vi "read caen.vi"(0 "VISA in":refnum<visa-resource-name>, 1 "Extended Delay":bool=TRUE, 11 "error in":errorcluster, 12 "First read time (ms)":u32=310, 13 "Short Loop Read Time (ms)":u32=150) -> (4 "VISA out":refnum<visa-resource-name>, 6 "Read string":string, 8 "Display array":string[][](array[string]), 10 "Location Cluster":T1, 14 "Display string":string, 15 "error out":errorcluster)   [LabVIEW 2018]
uses:
  location cluster.ctl
  <vilib>/Instr/_visa.llb/Select Event Type.ctl
  CAEN globals.vi
panel:
  out "Waveform Chart":i32(graph)
  out "HB":bool
  out "buffer":string
  out "Display":string[][](array[string])
  out "display error":errorcluster
  out "bytes at port":u32
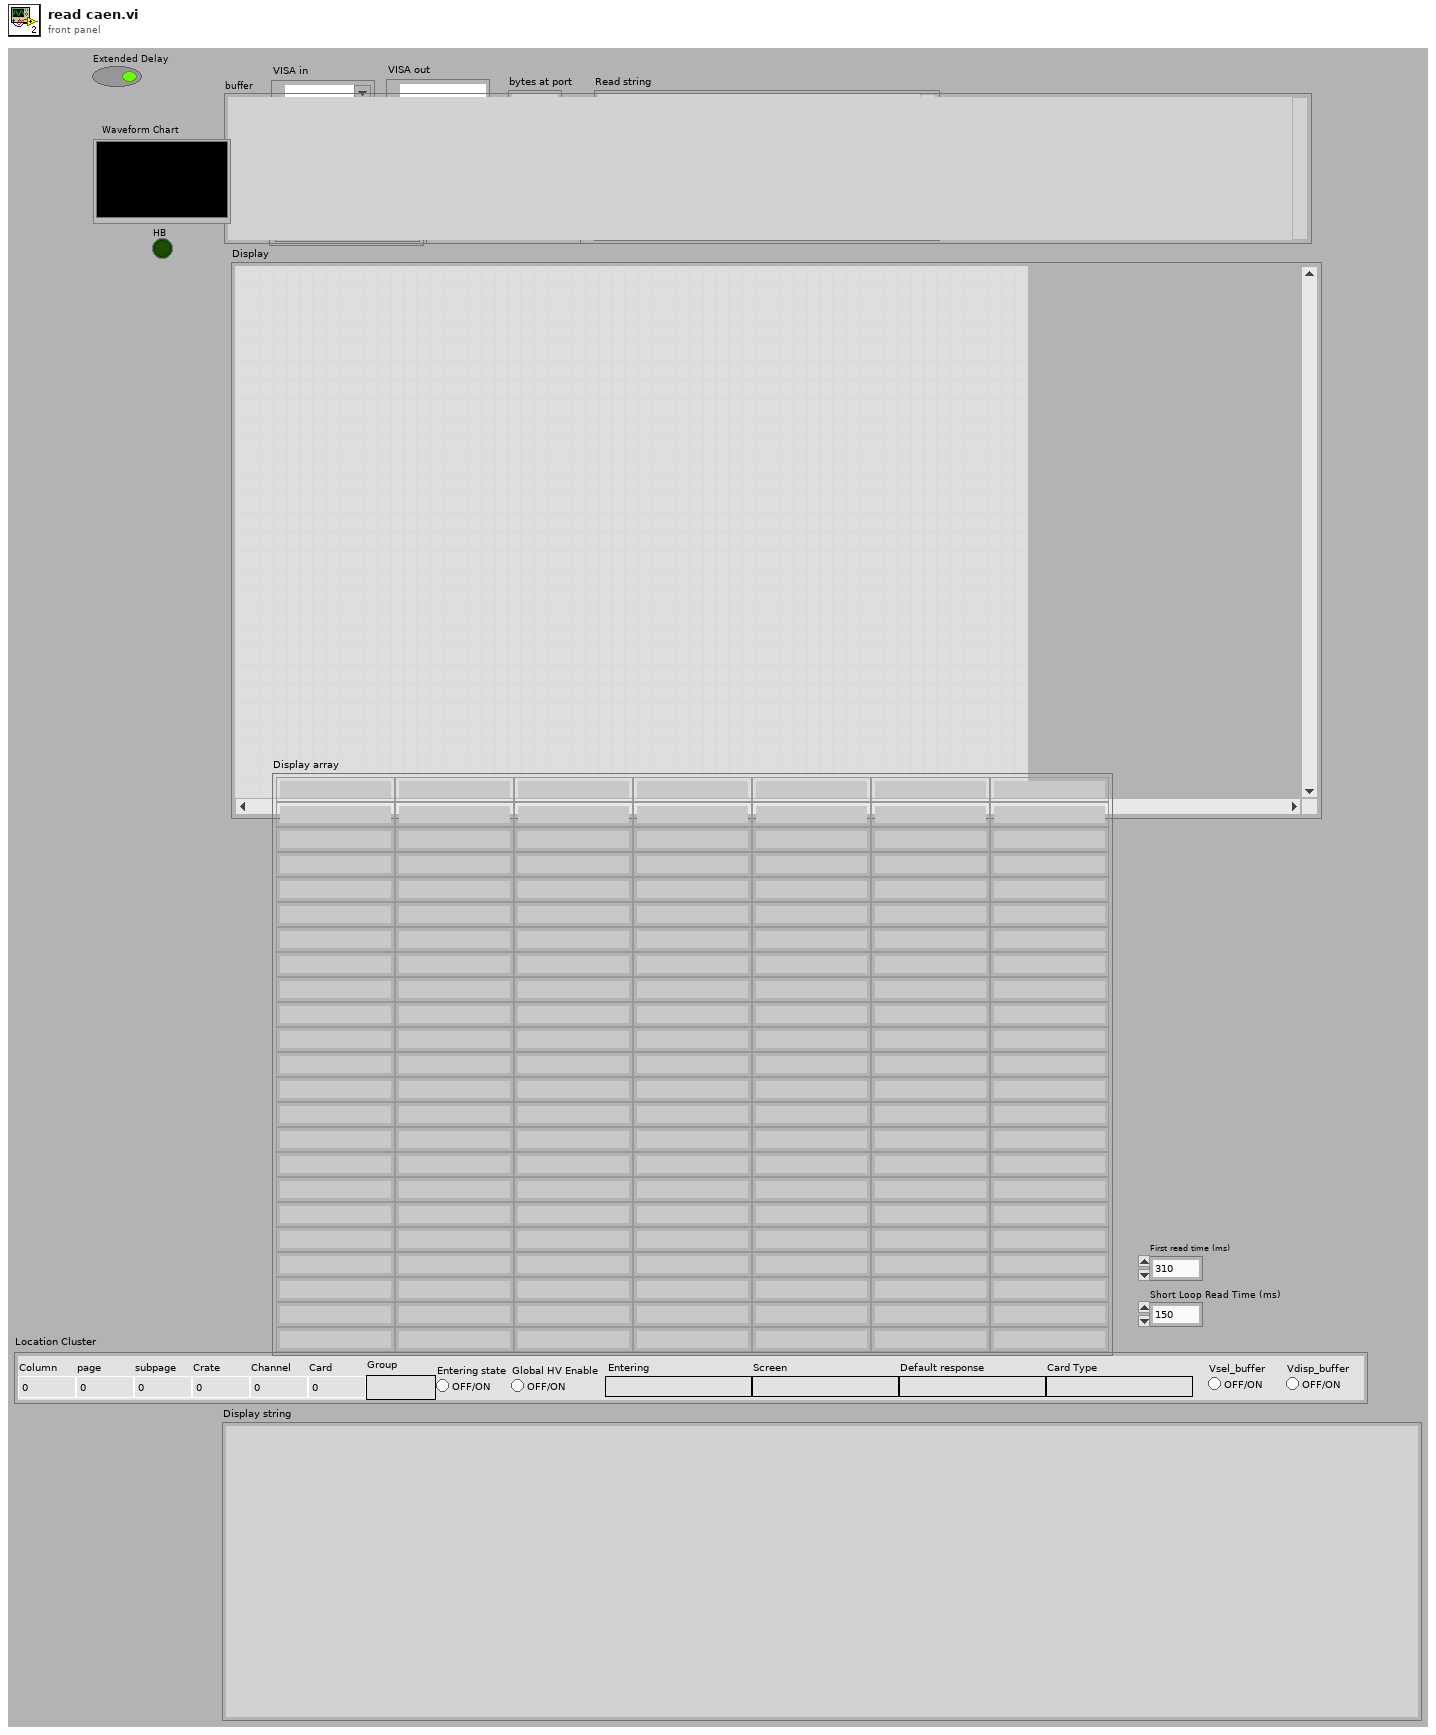
[diagram p1: front panel]
types:
  T1 = typedef "location cluster.ctl" = cluster{"Column":i32, "Card Type":string, "Channel":i32, "Card":i32, "Default response":string, "Entering":string, "Entering state":bool, "subpage":i32, "page":i32, "Crate":i32, "Screen":string, "Group":string, "Global HV Enable":bool, "Vsel_buffer":bool, "Vdisp_buffer":bool}
  T2 = typedef "Select Event Type.ctl" = u32
  T3 = cluster{"Bytes at Port":u32, "Serial Settings:Number of Bytes at Serial Port":u32}
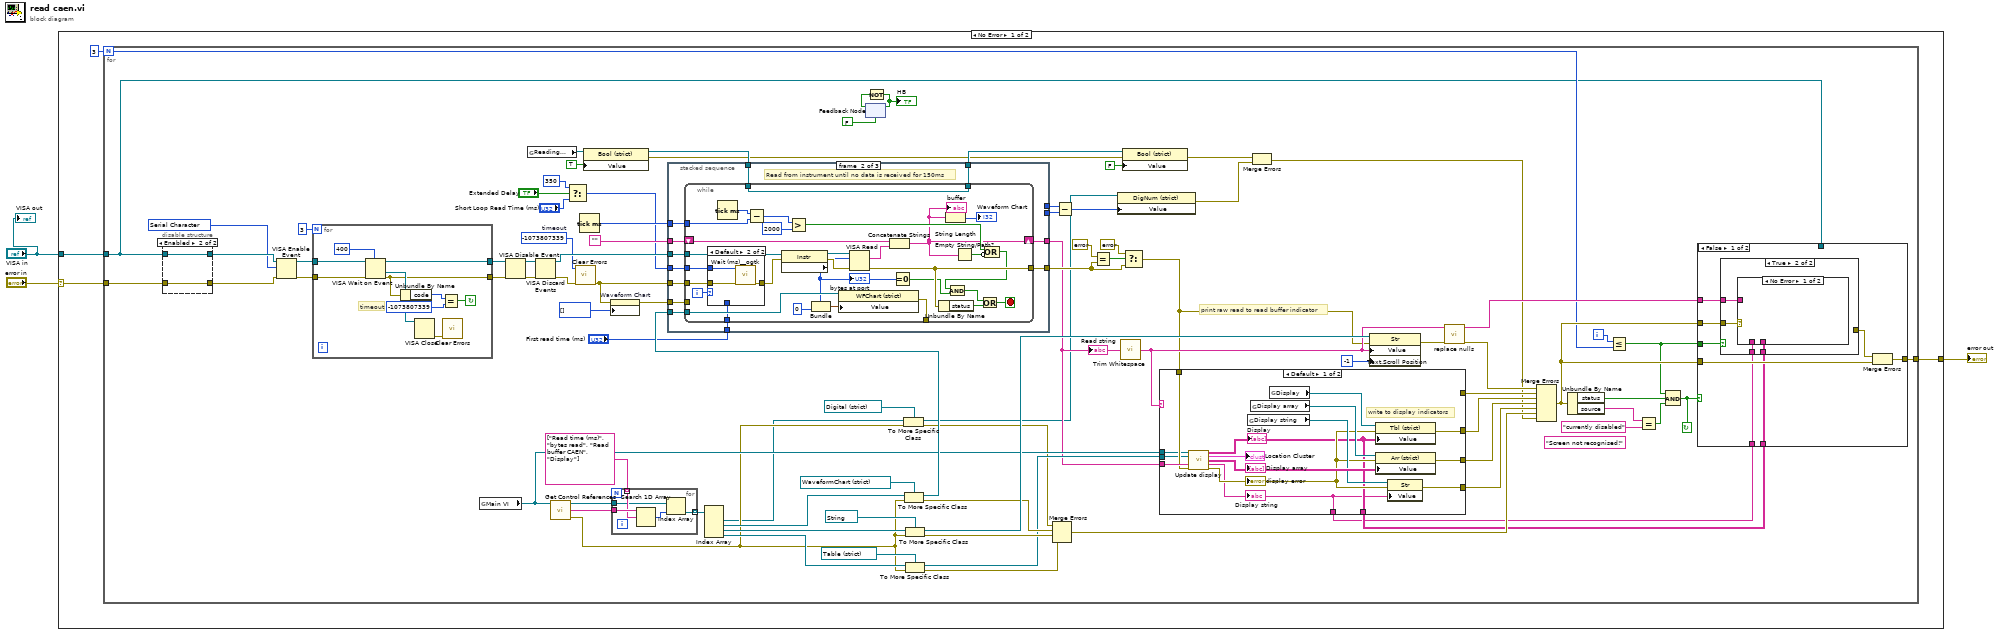
[diagram p0: block diagram]
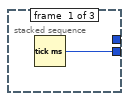
[diagram p2: hidden frame]
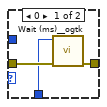
[diagram p3: hidden frame]
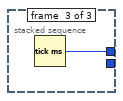
[diagram p4: hidden frame]
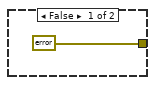
[diagram p5: hidden frame]
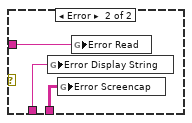
[diagram p6: hidden frame]
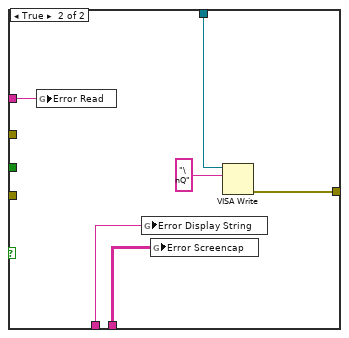
[diagram p7: hidden frame]
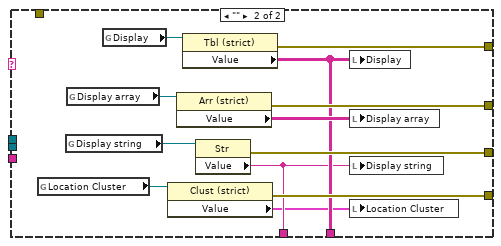
[diagram p8: hidden frame]
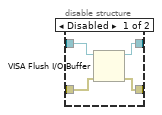
[diagram p9: hidden frame]
diagram:
  n1 = case shown="No Error" "error in" {
    selector: "error in" -> [w4 w218]
    tunnel: [w6 w218] -> w3
    tunnel: "VISA in" -> [w5 _]
    frame No Error {
      n2 = for {
        N: 3 -> [w26]
        tunnel: w4 -> [w74]
        tunnel: w5 -> [w8]
        tunnel: [w47] -> w6
        i -> [w27]
        stop <- w48 continue-if-true
        (unwired) "Screen not recognised!" ("y")
        w35 = -1073807339  # timeout
        w64 = T2 1073684533 items=["Service Request"=1073684491, "Trigger"=3221168138, "Clear"=1073684493, "VXI Signal"=1073684512, "VXI/VME Interrupt"=3221168161, "VXI/VME Sysfail"=1073684509, "VXI/VME Sysreset"=1073684510, "GPIB CIC"=1073684498, "GPIB Talk"=1073684499, "GPIB Listen"=1073684500, "PXI Interrupt"=1073684514, "Serial Break"=1073684515, "Serial TermChar"=1073684516, "Serial CTS"=1073684521, "Serial DSR"=1073684522, "Serial DCD"=1073684524, "Serial RI"=1073684526, "Serial Character"=1073684533, "USB Interrupt"=1073684535, "All Enabled"=1073709055] ("Event Type")
        # "print raw read to read buffer indicator"
        n3 = disable-structure shown="Enabled" {
          disable-tunnel: w8 -> [w210 w212]
          disable-tunnel: w74 -> [w209 w211]
          disable-tunnel: [w208 w212] -> w73
          disable-tunnel: [w207 w211] -> w72
          frame Disabled {
            n4 = VISA Flush I/O Buffer(VISA resource name=w210, error in (no error)=w209) -> (VISA resource name out=w208:refnum<visa-resource-name>, error out=w207:errorcluster)  [unwired: 1 in]
          }
          frame Enabled {
          }
        }
        n5 = VISA Enable Event(8:w72, 10:w64, 11:w73) -> (0:w42:errorcluster, 3:w43:refnum<visa-resource-name>)  [unwired: 1 in]
        n6 = for {
          N: 3 -> [_]
          tunnel: w42 -> [w156]
          tunnel: [w152] -> w37
          tunnel: w43 -> [w157]
          tunnel: [w153] -> w38
          stop <- w149 continue-if-true
          # "timeout"
          n7 = VISA Wait on Event(7:u32 400 ("milliseconds to wait"), 8:w156, 11:w157) -> (0:w152:errorcluster, 1:w155:refnum<visa-resource-name>, 3:w153:refnum<visa-resource-name>)  [unwired: 2 in, 1 out]
          n8 = Unbundle By Name(w152) -> ("code"=w151:i32)
          n9 = VISA Close(VISA resource name=w155) -> (error out=w154:errorcluster)  [unwired: 1 in]
          n10 = Equal?(x=w151, y=-1073807339) -> (x = y?=w149:bool)
          n11 = call <vilib>:"Clear Errors.vi"("error in (no error)"=w154) -> ()  [unwired: 5 in, 2 out]
        }
        n12 = global read "CAEN globals.vi" "Main VI"() -> (w76:refnum<vi>)
        n13 = VISA Disable Event(8:w37, 11:w38) -> (0:w40:errorcluster, 3:w39:refnum<visa-resource-name>)  [unwired: 2 in]
        n14 = global read "CAEN globals.vi" "Reading..."() -> (w63:refnum<vi>)
        n15 = VISA Discard Events(8:w40, 11:w39) -> (0:w36:errorcluster, 3:w71:refnum<visa-resource-name>)  [unwired: 2 in]
        n16 = call "Get Control References.vi"("This vi"=w76) -> ("error out"=w20:errorcluster, "Control Names"=w79:string[], "Controls[]"=w80:refnum<vi>[])  [unwired: 2 in]
        n17 = Select(t=u32 350 ("milliseconds to wait"), s="Extended Delay", f="Short Loop Read Time (ms)") -> (s? t:f=w44:u32)
        n18 = call <vilib>:"Clear Errors.vi"("error in (no error)"=w36, "specific error code to clear (0: all)"=w35) -> ("error out"=w67:errorcluster)  [unwired: 4 in, 1 out]
        n19 = Tick Count (ms)() -> (millisecond timer value=w96:u32)
        n20 = property class="Bool (strict)"(reference=w63, "Value"=TRUE ("x > y?")) -> (reference out=w62:refnum<vi>, error out=w58:errorcluster)  [unwired: 1 in]
        n21 = property on="Waveform Chart" class="WFChart (strict)"(error in=w67, "History Data"=i32[] []) -> (error out=w66:errorcluster)  [unwired: 1 in, 1 out]
        n22 = for {
          tunnel: w79 -> [w217]
          tunnel: string[] ["Read time (ms)", "bytes read", "Read buffer CAEN", "Display"] ("Array") -> [w216] mode=indexing
          tunnel: w80 -> [w215]
          tunnel: [w214] -> w95 mode=indexing
          n23 = Search 1D Array(1D array=w217, element=w216) -> (index of element=w213:i32)  [unwired: 1 in]
          n24 = Index Array(array=w215, index=w213) -> (element=w214:refnum<vi>)
        }
        n25 = Index Array(array=w95) -> (element #1=w19:refnum<vi>, element #2=w88:refnum<vi>, element #3=w93:refnum<vi>, element #4=w51:refnum<vi>)  [unwired: 4 in]
        n26 = feedback #1(FALSE ("x > y?")) -> (w69:bool)
        n27 = Not(x=w69) -> (.not. x?=w68:bool)
        "HB" <- w68
        n28 = feedback-in #1(w68) -> ()
        n29 = To More Specific Class(target class=refnum<vi> refnum ("Read time (ms)"), reference=w19, error in=w20) -> (specific class reference=w17:refnum<vi>, error out=w18:errorcluster)
        n30 = To More Specific Class(target class=refnum<vi> refnum ("bytes read"), reference=w88, error in=w20) -> (specific class reference=w87:refnum<vi>, error out=w89:errorcluster)
        n31 = stacked-sequence {
          tunnel: w96 -> [_ w110 _]
          tunnel: w87 -> [_ w109 _]
          tunnel: [_ w108 _] -> w83
          tunnel: w71 -> [_ w107 _]
          tunnel: w67 -> [_ w106 _]
          tunnel: w66 -> [_ w105 _]
          tunnel: w62 -> [_ w104 _]
          tunnel: [_ w103 _] -> w61
          tunnel: "" -> [_ w102 _]
          tunnel: w44 -> [_ w101 _]
          tunnel: [_ w100 _] -> w23
          tunnel: [w98 _ _] -> w12
          tunnel: [_ _ w147] -> w13
          tunnel: "First read time (ms)" -> [_ w99 _]
          frame #0 {
            n32 = Tick Count (ms)() -> (millisecond timer value=w98:u32)
          }
          frame #1 {
            # "Read from instrument until no data is received for 150ms"
            n33 = while {
              tunnel: w107 -> [w140]
              tunnel: [w134] -> w108
              shift-right: [w113] -> w100
              shift-left: w102 -> [w136]
              tunnel: w106 -> [w131]
              tunnel: w110 -> [w128]
              tunnel: w109 -> [w122]
              tunnel: [w121] -> _
              tunnel: w105 -> [_]
              tunnel: w104 -> [w115]
              tunnel: [w115] -> w103
              tunnel: w101 -> [w112]
              tunnel: w99 -> [w111]
              i -> [w114]
              stop <- w132 stop-if-true
              n34 = case shown="Default" w114 {
                tunnel: [w143 w146] -> w137
                tunnel: w131 -> [w142 w145]
                tunnel: w112 -> [_ w144]
                tunnel: w111 -> [w141 _]
                frame 0 {
                  n35 = call <userlib>:"Wait (ms)__ogtk.vi"("error in (no error)"=w142, "milliseconds to wait"=w141) -> ("error out"=w143:errorcluster)  [unwired: 8 in, 1 out]
                }
                frame Default {
                  n36 = call <userlib>:"Wait (ms)__ogtk.vi"("error in (no error)"=w145, "milliseconds to wait"=w144) -> ("error out"=w146:errorcluster)  [unwired: 8 in, 1 out]
                }
              }
              n37 = Tick Count (ms)() -> (millisecond timer value=w129:u32)
              n38 = Subtract(x=w129, y=w128) -> (x-y=w127:u32)
              n39 = property class="Instr"(reference=w140, error in=w137) -> (reference out=w138:refnum<visa-resource-name>, error out=w139:errorcluster, "Serial Settings:Number of Bytes at Serial Port"=w117:u32)
              "bytes at port" <- w117
              n40 = Greater?(x=w127, y=u32 2000) -> (0:w124:bool)
              n41 = Bundle("Bytes at Port"=w117, "Serial Settings:Number of Bytes at Serial Port"=u32 0) -> (w120:T3)  [unwired: 1 in]
              n42 = property class="WFChart (strict)"(reference=w122, "Value"=w120) -> (error out=w121:errorcluster)  [unwired: 1 in, 1 out]
              n43 = VISA Read(VISA resource name=w138, byte count=w117, error in (no error)=w139) -> (read buffer=w135:string, error out=w134:errorcluster)  [unwired: 2 out]
              n44 = Concatenate Strings(w136, w135) -> (w113:string)
              "buffer" <- w113
              n45 = Equal To 0?(x=w117) -> (x = 0?=w116:bool)
              n46 = Unbundle By Name(w134) -> ("status"=w133:bool)
              n47 = String Length(string=w113) -> (length=→"Waveform Chart":i32)
              n48 = Empty String/Path?(string/path=w113) -> (empty?=w125:bool)
              n49 = Compound Arithmetic op=OR(w124, invert w125) -> (w123:bool)
              n50 = Compound Arithmetic op=AND(w123, w116) -> (w130:bool)
              n51 = Or(x=w130, y=w133) -> (x .or. y?=w132:bool)
            }
          }
          frame #2 {
            n52 = Tick Count (ms)() -> (millisecond timer value=w147:u32)
          }
        }
        "Read string" <- w23
        n53 = To More Specific Class(target class=refnum<vi> refnum ("s? t:f"), reference=w93, error in=w20) -> (specific class reference=w90:refnum<vi>, error out=w92:errorcluster)
        n54 = To More Specific Class(target class=refnum<vi> refnum ("Display"), reference=w51, error in=w20) -> (specific class reference=w49:refnum<vi>, error out=w50:errorcluster)
        n55 = Merge Errors(w18, w89, w92, w50) -> (w82:errorcluster)
        n56 = Subtract(x=w13, y=w12) -> (x-y=w11:u32)
        n57 = Equal?(x=errorcluster {"status"=FALSE, "code"=1073676294, "source"="VISA Read in read.vi->read caen.vi"} ("error out 2"), y=w83) -> (x = y?=w85:bool)
        n58 = property class="DigNum (strict)"(reference=w17, "Value"=w11) -> (error out=w16:errorcluster)  [unwired: 1 in, 1 out]
        n59 = call <vilib>:"Trim Whitespace.vi"("string"=w23) -> ("trimmed string"=w29:string)  [unwired: 1 in]
        n60 = property class="Bool (strict)"(reference=w61, error in=w58, "Value"=FALSE ("x > y?")) -> (error out=w15:errorcluster)  [unwired: 1 out]
        n61 = Select(t=errorcluster {"status"=FALSE, "code"=0, "source"=""}, s=w85, f=w83) -> (s? t:f=w22:errorcluster)
        n62 = case shown="Default" w29 {
          tunnel: w23 -> [w194 _]
          tunnel: w22 -> [w192 _]
          tunnel: w49 -> [w191 _]
          tunnel: [w188 w200] -> w78
          tunnel: [w187 w199] -> w77
          tunnel: w76 -> [w185 _]
          tunnel: [w184 w201] -> w75
          tunnel: [w181 w197] -> w34
          tunnel: [_ w198] -> w33
          tunnel: [w180 w196] -> w24
          frame Default {
            # "write to display indicators"
            n63 = call "Update display.vi"("This VI"=w185, "Display"=w191, "input"=w194, "error in"=w192) -> ("Display out"=w181:string[][], "Location Cluster out"=→"Location Cluster":T1, "Display array"=w189:string[][], "Display string"=w180:string, "Error Out"=w182:errorcluster)  [unwired: 7 in]
            "display error" <- w182
            "Display" <- w181
            "Display array" <- w189
            "Display string" <- w180
            n64 = global read "CAEN globals.vi" "Display string"() -> (w183:refnum<vi>)
            n65 = global read "CAEN globals.vi" "Display array"() -> (w190:refnum<vi>)
            n66 = global read "CAEN globals.vi" "Display"() -> (w186:refnum<vi>)
            n67 = property class="Tbl (strict)"(reference=w186, error in=w182, "Value"=w181) -> (error out=w187:errorcluster)  [unwired: 1 out]
            n68 = property class="Arr (strict)"(reference=w190, error in=w182, "Value"=w189) -> (error out=w188:errorcluster)  [unwired: 1 out]
            n69 = property class="Str"(reference=w183, error in=w182, "Value"=w180) -> (error out=w184:errorcluster)  [unwired: 1 out]
          }
          frame "" {
            n70 = global read "CAEN globals.vi" "Location Cluster"() -> (w202:refnum<vi>)
            n71 = global read "CAEN globals.vi" "Display string"() -> (w204:refnum<vi>)
            n72 = global read "CAEN globals.vi" "Display array"() -> (w206:refnum<vi>)
            n73 = global read "CAEN globals.vi" "Display"() -> (w205:refnum<vi>)
            n74 = property class="Clust (strict)"(reference=w202) -> (error out=w201:errorcluster, "Value"=w195:T1)  [unwired: 1 in, 1 out]
            n75 = property class="Arr (strict)"(reference=w206) -> (error out=w199:errorcluster, "Value"=w203:string[][])  [unwired: 1 in, 1 out]
            n76 = property class="Tbl (strict)"(reference=w205) -> (error out=w198:errorcluster, "Value"=w197:string[][])  [unwired: 1 in, 1 out]
            n77 = property class="Str"(reference=w204) -> (error out=w200:errorcluster, "Value"=w196:string)  [unwired: 1 in, 1 out]
            n78 = local write "Display"(w197) -> ()
            n79 = local write "Display array"(w203) -> ()
            n80 = local write "Display string"(w196) -> ()
            n81 = local write "Location Cluster"(w195) -> ()
          }
        }
        n82 = Merge Errors(w15, w16) -> (w14:errorcluster)
        n83 = property class="Str"(reference=w90, error in=w22, "Value"=w29, "Text.Scroll Position"=-1) -> (error out=w31:errorcluster)  [unwired: 1 out]
        n84 = call "replace nulls.vi"("error in (no error)"=w31, "read buffer"=w29) -> ("error out"=w30:errorcluster, "result string"=w28:string)  [unwired: 8 in]
        n85 = Merge Errors(w30, w33, w77, w78, w75, w82, w14) -> (w32:errorcluster)
        n86 = Unbundle By Name(w32) -> ("status"=w56:bool, "source"=w54:string)
        n87 = Less Or Equal?(x=w27, y=w26) -> (x <= y?=w25:bool)
        n88 = Equal?(x=w54, y="currently disabled") -> (x = y?=w55:bool)
        n89 = Compound Arithmetic op=AND(w25, w56, w55) -> (w48:bool)
        n90 = case shown="False" w48 {
          tunnel: w8 -> [_ w179]
          tunnel: [w165 w177] -> w47
          tunnel: w32 -> [w164 _]
          tunnel: w25 -> [w160 _]
          tunnel: w34 -> [w161 w176]
          tunnel: w28 -> [w162 w175]
          tunnel: w32 -> [w163 _]
          tunnel: w24 -> [w158 w174]
          frame False {
            n91 = case shown="True" w160 {
              tunnel: w164 -> [_ w170]
              tunnel: w162 -> [_ w169]
              tunnel: w161 -> [_ w168]
              tunnel: [errorcluster {"status"=TRUE, "code"=0, "source"="Screen not recognised!"} ("error IO") _] -> w159
              tunnel: w158 -> [_ w167]
              frame False {
              }
              frame True {
                n92 = case shown="No Error" w170 {
                  tunnel: w169 -> [_ w173]
                  tunnel: w168 -> [_ w172]
                  tunnel: w167 -> [_ w171]
                  frame No Error {
                  }
                  frame Error {
                    n93 = global write "CAEN globals.vi" "Error Display String"(w171) -> ()
                    n94 = global write "CAEN globals.vi" "Error Screencap"(w172) -> ()
                    n95 = global write "CAEN globals.vi" "Error Read"(w173) -> ()
                  }
                }
              }
            }
            n96 = Merge Errors(w159, w163) -> (w165:errorcluster)
          }
          frame True {
            n97 = global write "CAEN globals.vi" "Error Read"(w175) -> ()
            n98 = global write "CAEN globals.vi" "Error Display String"(w174) -> ()
            n99 = global write "CAEN globals.vi" "Error Screencap"(w176) -> ()
            n100 = VISA Write(VISA resource name=w179, write buffer="\nQ") -> (error out=w177:errorcluster)  [unwired: 1 in, 2 out]
          }
        }
      }
    }
    frame Error {
    }
  }
  "error out" <- w3
  "VISA out" <- "VISA in"
